vi "GrabberWheels Controller.vi"(8 "error in (no error)":errorcluster, 9 "GW Spit Out":bool, 10 "GW Half Speed Pickup":bool, 11 "GW Full Speed Pickup":bool) -> (0 "error out":errorcluster)   [LabVIEW 2013]
uses:
  Systems/GrabberWheels/GrabberWheels.lvclass
  Robot Global Data.vi
  Commands/GW-PickUp-Command/GW-PickUp-Cmd.lvclass
  Commands/GW-Stop-Command/GW-Stop-Cmd.lvclass
  Commands/GW-PickUp(Half)-Command/GW-PickUp(Half)-Cmd.lvclass
  Commands/GW-SpitOut-Command/GW-SpitOut-Cmd.lvclass
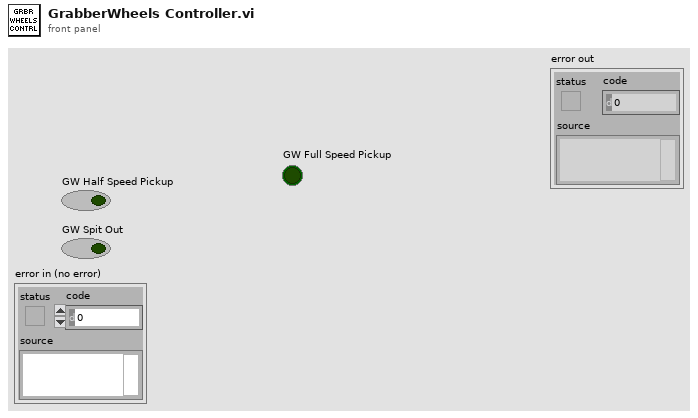
[diagram p1: front panel]
types:
  T1 = typedef "Semaphore RefNum" = refnum<k1>
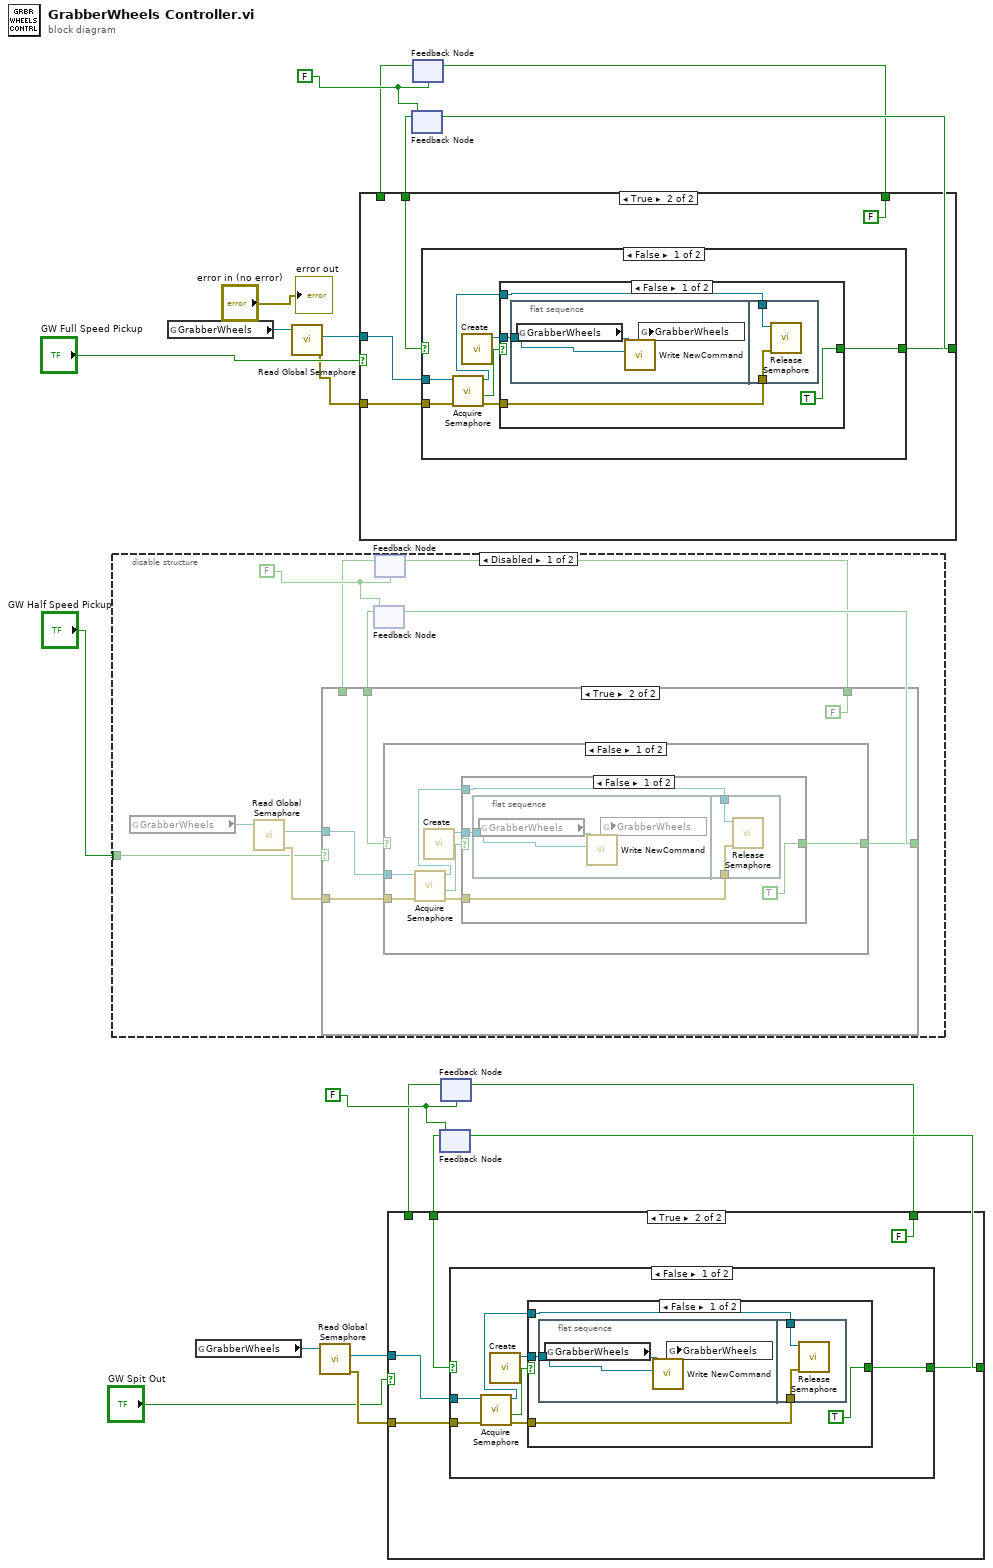
[diagram p0: block diagram]
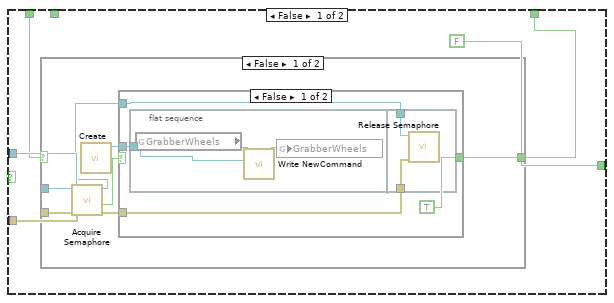
[diagram p2: hidden frame]
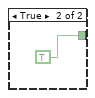
[diagram p3: hidden frame]
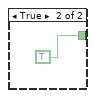
[diagram p5: hidden frame]
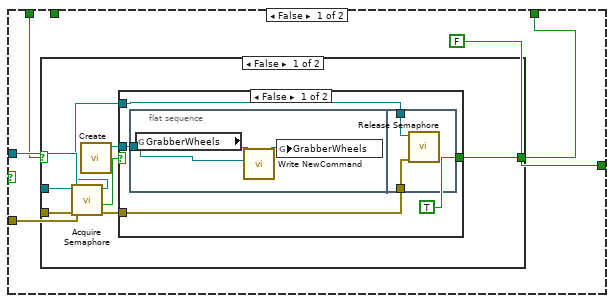
[diagram p8: hidden frame]
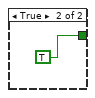
[diagram p9: hidden frame]
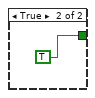
[diagram p11: hidden frame]
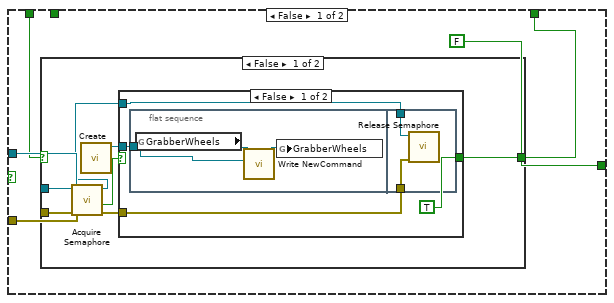
[diagram p13: hidden frame]
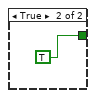
[diagram p14: hidden frame]
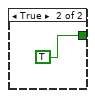
[diagram p16: hidden frame]
diagram:
  w10 = FALSE
  w19 = FALSE
  n1 = disable-structure shown="Disabled" {
    disable-tunnel: "GW Half Speed Pickup" -> [w21 _]
    frame Disabled {
      w29 = FALSE
      n2 = global read "Robot Global Data.vi" "GrabberWheels"() -> (w26:refnum<class "GrabberWheels.lvclass">)
      n3 = call-dynamic "Read Global Semaphore.vi"("System in"=w26) -> ("error out"=w24:errorcluster, "semaphore"=w25:T1)  [unwired: 8 in, 1 out]
      n4 = feedback #1(w29) -> (w28:bool)
      n5 = feedback #2(w29) -> (w22:bool)
      n6 = case shown="True" w21 {
        tunnel: w28 -> [_ w57]
        tunnel: [FALSE w56] -> w27
        tunnel: w25 -> [w34 w55]
        tunnel: w24 -> [w33 w54]
        tunnel: [w32 FALSE] -> w23
        tunnel: w22 -> [w30 _]
        frame False {
          n7 = case shown="False" w30 {
            selector: w30 -> [_ w52]
            tunnel: [w35 w52] -> w32
            tunnel: w34 -> [w41 _]
            tunnel: w33 -> [w40 _]
            frame False {
              n8 = call <vilib>:"Acquire Semaphore.vi"("error in (no error)"=w40, "semaphore"=w41) -> ("error out"=w39:errorcluster, "timed out"=w36:bool, "semaphore out"=w38:T1)  [unwired: 3 in]
              n9 = call "Create.vi"() -> ("GW-Stop-Cmd out"=w37:refnum<class "GW-Stop-Cmd.lvclass">)  [unwired: 10 in, 1 out]
              n10 = case shown="False" w36 {
                tunnel: w39 -> [w45 _]
                tunnel: w38 -> [w44 _]
                tunnel: w37 -> [w43 _]
                tunnel: [TRUE TRUE] -> w35
                frame False {
                  n11 = flat-sequence {
                    tunnel: w43 -> [w46]
                    tunnel: w45 -> [w50]
                    tunnel: w44 -> [w49]
                    frame #0 {
                      n12 = global read "Robot Global Data.vi" "GrabberWheels"() -> (w48:refnum<class "GrabberWheels.lvclass">)
                      n13 = call-dynamic "Write NewCommand.vi"("Command.lvclass"=w46, "System in"=w48) -> ("System out"=w47:refnum<class "GrabberWheels.lvclass">)  [unwired: 8 in, 1 out]
                      n14 = global write "Robot Global Data.vi" "GrabberWheels"(w47) -> ()
                    }
                    frame #1 {
                      n15 = call <vilib>:"Release Semaphore.vi"("error in (no error)"=w50, "semaphore"=w49) -> ()  [unwired: 4 in, 2 out]
                    }
                  }
                }
                frame True {
                }
              }
            }
            frame True {
            }
          }
        }
        frame True {
          n16 = case shown="False" w57 {
            selector: w57 -> [_ w75]
            tunnel: [w58 w75] -> w56
            tunnel: w55 -> [w64 _]
            tunnel: w54 -> [w63 _]
            frame False {
              n17 = call <vilib>:"Acquire Semaphore.vi"("error in (no error)"=w63, "semaphore"=w64) -> ("error out"=w62:errorcluster, "timed out"=w59:bool, "semaphore out"=w61:T1)  [unwired: 3 in]
              n18 = call "Create.vi"() -> ("GW-PickUp(Half)-Cmd.lvclass"=w60:refnum<class "GW-PickUp(Half)-Cmd.lvclass">)  [unwired: 10 in, 1 out]
              n19 = case shown="False" w59 {
                tunnel: w62 -> [w68 _]
                tunnel: w61 -> [w67 _]
                tunnel: w60 -> [w66 _]
                tunnel: [TRUE TRUE] -> w58
                frame False {
                  n20 = flat-sequence {
                    tunnel: w66 -> [w69]
                    tunnel: w68 -> [w73]
                    tunnel: w67 -> [w72]
                    frame #0 {
                      n21 = global read "Robot Global Data.vi" "GrabberWheels"() -> (w71:refnum<class "GrabberWheels.lvclass">)
                      n22 = call-dynamic "Write NewCommand.vi"("Command.lvclass"=w69, "System in"=w71) -> ("System out"=w70:refnum<class "GrabberWheels.lvclass">)  [unwired: 8 in, 1 out]
                      n23 = global write "Robot Global Data.vi" "GrabberWheels"(w70) -> ()
                    }
                    frame #1 {
                      n24 = call <vilib>:"Release Semaphore.vi"("error in (no error)"=w73, "semaphore"=w72) -> ()  [unwired: 4 in, 2 out]
                    }
                  }
                }
                frame True {
                }
              }
            }
            frame True {
            }
          }
        }
      }
      n25 = feedback-in #1(w27) -> ()
      n26 = feedback-in #2(w23) -> ()
    }
    frame Enabled {
    }
  }
  n27 = global read "Robot Global Data.vi" "GrabberWheels"() -> (w16:refnum<class "GrabberWheels.lvclass">)
  n28 = global read "Robot Global Data.vi" "GrabberWheels"() -> (w7:refnum<class "GrabberWheels.lvclass">)
  n29 = call-dynamic "Read Global Semaphore.vi"("System in"=w16) -> ("error out"=w14:errorcluster, "semaphore"=w15:T1)  [unwired: 8 in, 1 out]
  n30 = call-dynamic "Read Global Semaphore.vi"("System in"=w7) -> ("error out"=w5:errorcluster, "semaphore"=w6:T1)  [unwired: 8 in, 1 out]
  n31 = feedback #3(w19) -> (w18:bool)
  n32 = feedback #4(w19) -> (w12:bool)
  n33 = case shown="True" "GW Full Speed Pickup" {
    tunnel: w18 -> [_ w103]
    tunnel: [FALSE w102] -> w17
    tunnel: w15 -> [w80 w101]
    tunnel: w14 -> [w79 w100]
    tunnel: [w78 FALSE] -> w13
    tunnel: w12 -> [w76 _]
    frame False {
      n34 = case shown="False" w76 {
        selector: w76 -> [_ w98]
        tunnel: [w81 w98] -> w78
        tunnel: w80 -> [w87 _]
        tunnel: w79 -> [w86 _]
        frame False {
          n35 = call <vilib>:"Acquire Semaphore.vi"("error in (no error)"=w86, "semaphore"=w87) -> ("error out"=w85:errorcluster, "timed out"=w82:bool, "semaphore out"=w84:T1)  [unwired: 3 in]
          n36 = call "Create.vi"() -> ("GW-Stop-Cmd out"=w83:refnum<class "GW-Stop-Cmd.lvclass">)  [unwired: 10 in, 1 out]
          n37 = case shown="False" w82 {
            tunnel: w85 -> [w91 _]
            tunnel: w84 -> [w90 _]
            tunnel: w83 -> [w89 _]
            tunnel: [TRUE TRUE] -> w81
            frame False {
              n38 = flat-sequence {
                tunnel: w89 -> [w92]
                tunnel: w91 -> [w96]
                tunnel: w90 -> [w95]
                frame #0 {
                  n39 = global read "Robot Global Data.vi" "GrabberWheels"() -> (w94:refnum<class "GrabberWheels.lvclass">)
                  n40 = call-dynamic "Write NewCommand.vi"("Command.lvclass"=w92, "System in"=w94) -> ("System out"=w93:refnum<class "GrabberWheels.lvclass">)  [unwired: 8 in, 1 out]
                  n41 = global write "Robot Global Data.vi" "GrabberWheels"(w93) -> ()
                }
                frame #1 {
                  n42 = call <vilib>:"Release Semaphore.vi"("error in (no error)"=w96, "semaphore"=w95) -> ()  [unwired: 4 in, 2 out]
                }
              }
            }
            frame True {
            }
          }
        }
        frame True {
        }
      }
    }
    frame True {
      n43 = case shown="False" w103 {
        selector: w103 -> [_ w121]
        tunnel: [w104 w121] -> w102
        tunnel: w101 -> [w110 _]
        tunnel: w100 -> [w109 _]
        frame False {
          n44 = call <vilib>:"Acquire Semaphore.vi"("error in (no error)"=w109, "semaphore"=w110) -> ("error out"=w108:errorcluster, "timed out"=w105:bool, "semaphore out"=w107:T1)  [unwired: 3 in]
          n45 = call "Create.vi"() -> ("GW-PickUp-Cmd out"=w106:refnum<class "GW-PickUp-Cmd.lvclass">)  [unwired: 10 in, 1 out]
          n46 = case shown="False" w105 {
            tunnel: w108 -> [w114 _]
            tunnel: w107 -> [w113 _]
            tunnel: w106 -> [w112 _]
            tunnel: [TRUE TRUE] -> w104
            frame False {
              n47 = flat-sequence {
                tunnel: w112 -> [w115]
                tunnel: w114 -> [w119]
                tunnel: w113 -> [w118]
                frame #0 {
                  n48 = global read "Robot Global Data.vi" "GrabberWheels"() -> (w117:refnum<class "GrabberWheels.lvclass">)
                  n49 = call-dynamic "Write NewCommand.vi"("Command.lvclass"=w115, "System in"=w117) -> ("System out"=w116:refnum<class "GrabberWheels.lvclass">)  [unwired: 8 in, 1 out]
                  n50 = global write "Robot Global Data.vi" "GrabberWheels"(w116) -> ()
                }
                frame #1 {
                  n51 = call <vilib>:"Release Semaphore.vi"("error in (no error)"=w119, "semaphore"=w118) -> ()  [unwired: 4 in, 2 out]
                }
              }
            }
            frame True {
            }
          }
        }
        frame True {
        }
      }
    }
  }
  n52 = feedback-in #3(w17) -> ()
  n53 = feedback-in #4(w13) -> ()
  n54 = feedback #5(w10) -> (w9:bool)
  n55 = feedback #6(w10) -> (w3:bool)
  n56 = case shown="True" "GW Spit Out" {
    tunnel: w9 -> [_ w149]
    tunnel: [FALSE w148] -> w8
    tunnel: w6 -> [w126 w147]
    tunnel: w5 -> [w125 w146]
    tunnel: [w124 FALSE] -> w4
    tunnel: w3 -> [w122 _]
    frame False {
      n57 = case shown="False" w122 {
        selector: w122 -> [_ w144]
        tunnel: [w127 w144] -> w124
        tunnel: w126 -> [w133 _]
        tunnel: w125 -> [w132 _]
        frame False {
          n58 = call <vilib>:"Acquire Semaphore.vi"("error in (no error)"=w132, "semaphore"=w133) -> ("error out"=w131:errorcluster, "timed out"=w128:bool, "semaphore out"=w130:T1)  [unwired: 3 in]
          n59 = call "Create.vi"() -> ("GW-Stop-Cmd out"=w129:refnum<class "GW-Stop-Cmd.lvclass">)  [unwired: 10 in, 1 out]
          n60 = case shown="False" w128 {
            tunnel: w131 -> [w137 _]
            tunnel: w130 -> [w136 _]
            tunnel: w129 -> [w135 _]
            tunnel: [TRUE TRUE] -> w127
            frame False {
              n61 = flat-sequence {
                tunnel: w135 -> [w138]
                tunnel: w137 -> [w142]
                tunnel: w136 -> [w141]
                frame #0 {
                  n62 = global read "Robot Global Data.vi" "GrabberWheels"() -> (w140:refnum<class "GrabberWheels.lvclass">)
                  n63 = call-dynamic "Write NewCommand.vi"("Command.lvclass"=w138, "System in"=w140) -> ("System out"=w139:refnum<class "GrabberWheels.lvclass">)  [unwired: 8 in, 1 out]
                  n64 = global write "Robot Global Data.vi" "GrabberWheels"(w139) -> ()
                }
                frame #1 {
                  n65 = call <vilib>:"Release Semaphore.vi"("error in (no error)"=w142, "semaphore"=w141) -> ()  [unwired: 4 in, 2 out]
                }
              }
            }
            frame True {
            }
          }
        }
        frame True {
        }
      }
    }
    frame True {
      n66 = case shown="False" w149 {
        selector: w149 -> [_ w167]
        tunnel: [w150 w167] -> w148
        tunnel: w147 -> [w156 _]
        tunnel: w146 -> [w155 _]
        frame False {
          n67 = call <vilib>:"Acquire Semaphore.vi"("error in (no error)"=w155, "semaphore"=w156) -> ("error out"=w154:errorcluster, "timed out"=w151:bool, "semaphore out"=w153:T1)  [unwired: 3 in]
          n68 = call "Create.vi"() -> ("GW-SpitOut-Cmd out"=w152:refnum<class "GW-SpitOut-Cmd.lvclass">)  [unwired: 10 in, 1 out]
          n69 = case shown="False" w151 {
            tunnel: w154 -> [w160 _]
            tunnel: w153 -> [w159 _]
            tunnel: w152 -> [w158 _]
            tunnel: [TRUE TRUE] -> w150
            frame False {
              n70 = flat-sequence {
                tunnel: w158 -> [w161]
                tunnel: w160 -> [w165]
                tunnel: w159 -> [w164]
                frame #0 {
                  n71 = global read "Robot Global Data.vi" "GrabberWheels"() -> (w163:refnum<class "GrabberWheels.lvclass">)
                  n72 = call-dynamic "Write NewCommand.vi"("Command.lvclass"=w161, "System in"=w163) -> ("System out"=w162:refnum<class "GrabberWheels.lvclass">)  [unwired: 8 in, 1 out]
                  n73 = global write "Robot Global Data.vi" "GrabberWheels"(w162) -> ()
                }
                frame #1 {
                  n74 = call <vilib>:"Release Semaphore.vi"("error in (no error)"=w165, "semaphore"=w164) -> ()  [unwired: 4 in, 2 out]
                }
              }
            }
            frame True {
            }
          }
        }
        frame True {
        }
      }
    }
  }
  n75 = feedback-in #5(w8) -> ()
  n76 = feedback-in #6(w4) -> ()
  "error out" <- "error in (no error)"
